vi "HP Data Type List.vi"(11 "HP Events Clust Refnum":refnum<vi>) -> (0 "error out":errorcluster, 3 "Data Type List":string[](array[string]))   [LabVIEW 2016, in "M1M3SupportEUI_Views.lvlib"]
uses:
  M1M3SupportEUI_Views.lvlib
  Typedefs/HP Events.ctl
  SALLV_m1m3/DataTypes/logevent_HardpointActuatorInfo.ctl
  SALLV_m1m3/DataTypes/logevent_HardpointActuatorState.ctl
  SALLV_m1m3/DataTypes/logevent_HardpointActuatorWarning.ctl
  SALLV_m1m3/DataTypes/logevent_HardpointMonitorInfo.ctl
  SALLV_m1m3/DataTypes/logevent_HardpointMonitorState.ctl
  SALLV_m1m3/DataTypes/logevent_HardpointMonitorWarning.ctl
  SALLV_m1m3/SALLV_m1m3.lvlib
  Typedefs/M1M3SupportEUI_TypeDefs.lvlib
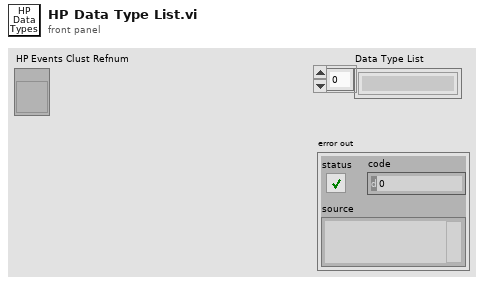
[diagram p1: front panel]
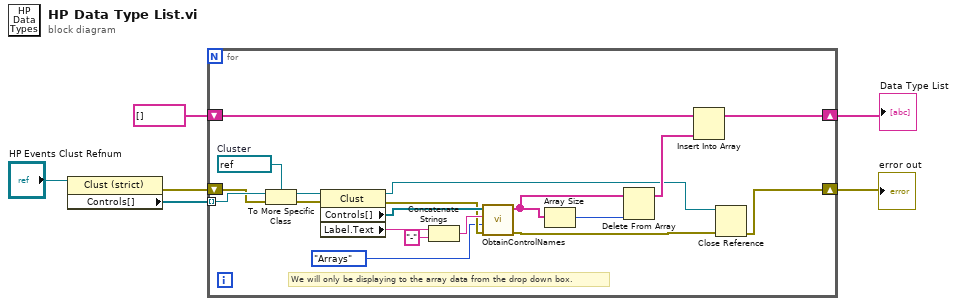
[diagram p0: block diagram]
diagram:
  n1 = property class="Clust (strict)"(reference="HP Events Clust Refnum") -> (error out=w4:errorcluster, "Controls[]"=w5:refnum<vi>[])  [unwired: 1 in, 1 out]
  n2 = for {
    tunnel: w5 -> [w25] mode=indexing
    shift-right: [w9] -> w3
    shift-left: w4 -> [w24]
    shift-right: [w12] -> w1
    shift-left: string[] [] -> [w14]
    w23 = refnum<vi> refnum  # Cluster
    # "We will only be displaying to the array data from the drop down box."
    n3 = To More Specific Class(target class=w23, reference=w25, error in=w24) -> (specific class reference=w22:refnum<vi>, error out=w21:errorcluster)
    n4 = property class="Clust"(reference=w22, error in=w21) -> (reference out=w8:refnum<vi>, error out=w11:errorcluster, "Controls[]"=w17:refnum<vi>[], "Label.Text"=w19:string)
    n5 = Concatenate Strings(w19, "-" ("string")) -> (w18:string)
    n6 = call "ObtainControlNames.vi"("error in (no error)"=w11, "ControlNameTypes"=enum16{"ALL", "Arrays", "SingleValues"}."Arrays", "AddedPrefix"=w18, "ControlRefnumArray"=w17) -> ("error out"=w10:errorcluster, "ControlNamesArray"=w16:string[])  [unwired: 6 in]
    n7 = Array Size(array=w16) -> (size(s)=w15:i32)
    n8 = Delete From Array(array=w16, index=w15) -> (array with subset deleted=w13:string[])  [unwired: 1 in, 1 out]
    n9 = Insert Into Array(array=w14, new element=w13) -> (w12:string[])  [unwired: 1 in]
    n10 = Close Reference(reference=w8, error in (no error)=w10) -> (error out=w9:errorcluster)
  }
  "Data Type List" <- w1
  "error out" <- w3
